vi "Get object by name.vi"(8 "error in (no error)":errorcluster, 10 "path":path, 11 "Folder in":refnum<class "Folder.lvclass">) -> (0 "error out":errorcluster, 1 "Found":bool, 2 "Object":refnum<class "system object.lvclass">, 3 "Folder out":refnum<class "Folder.lvclass">)   [LabVIEW 2020, in "Folder.lvclass"]
uses:
  Folder.lvclass
  system object/system object.lvclass
  Folder.lvclass/Folder.ctl
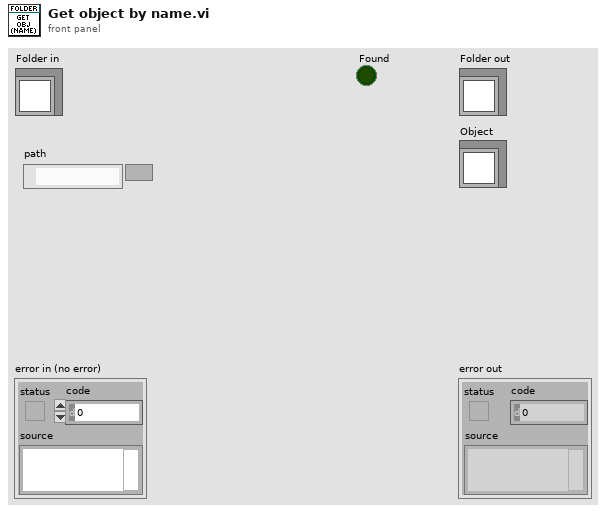
[diagram p1: front panel]
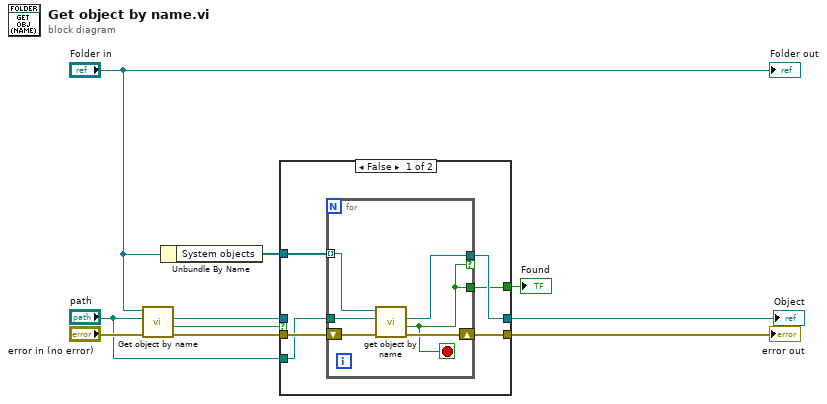
[diagram p0: block diagram]
diagram:
  n1 = call-parent "Get object by name.vi"("error in (no error)"="error in (no error)", "Name"="path", "system object in"="Folder in") -> ("error out"=w6:errorcluster, "Found"=w9:bool, "Target object"=w8:refnum<class "system object.lvclass">)  [unwired: 5 in, 1 out]
  n2 = Unbundle By Name("Folder in") -> ("System objects"=w7:refnum<class "system object.lvclass">[])
  n3 = case shown="False" w9 {
    selector: w9 -> [_ w23]
    tunnel: w8 -> [_ w25]
    tunnel: w7 -> [w16 _]
    tunnel: [w15 w25] -> w3
    tunnel: w6 -> [w14 w24]
    tunnel: [w13 w24] -> w5
    tunnel: [w12 w23] -> w2
    tunnel: "path" -> [w11 _]
    frame False {
      n4 = for {
        tunnel: w16 -> [w22] mode=indexing
        tunnel: [w19] -> w15 if=w18
        shift-right: [w20] -> w13
        shift-left: w14 -> [w21]
        tunnel: [w18] -> w12
        tunnel: w11 -> [w17]
        stop <- w18 stop-if-true
        n5 = call-dynamic "get object by name.vi"("error in (no error)"=w21, "Name"=w17, "system object in"=w22) -> ("error out"=w20:errorcluster, "Found"=w18:bool, "Target object"=w19:refnum<class "system object.lvclass">)  [unwired: 5 in, 1 out]
      }
    }
    frame True {
    }
  }
  "error out" <- w5
  "Object" <- w3
  "Found" <- w2
  "Folder out" <- "Folder in"
